vi "SetMotorType.vi"(0 "CmdLib In":refnum<k24>, 5 "DeviceKey In":string, 7 "Motor":i32, 9 "Motor Type":i32(ring) items=["NoMotor", "Undefined", "Tiny", "Standard"], 11 "error in (no error)":errorcluster) -> (4 "CmdLib Out":refnum<k24>, 8 "DeviceKey Out":string, 15 "error out":errorcluster)   [LabVIEW 2013]
uses:
  C:/Users/Saffmanlab/Documents/git/CsPyController/labview/cesium_controller/PicoMotor/NewFocus8742/CmdLib.dll
  CmdLib.dll
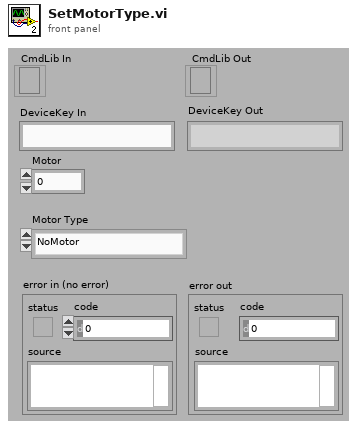
[diagram p1: front panel]
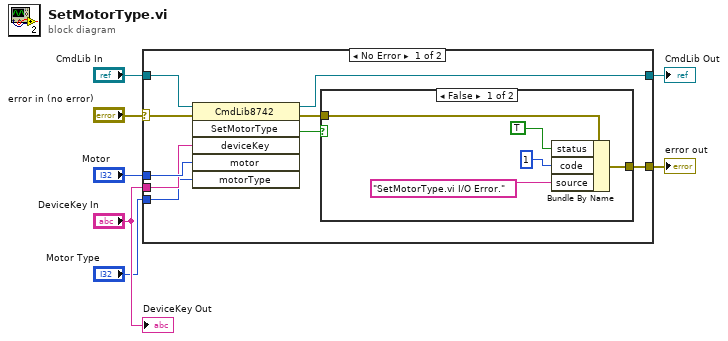
[diagram p0: block diagram]
diagram:
  n1 = case shown="No Error" "error in (no error)" {
    selector: "error in (no error)" -> [w12 w23]
    tunnel: "CmdLib In" -> [w16 w24]
    tunnel: [w15 w24] -> w6
    tunnel: "Motor" -> [w14 _]
    tunnel: "DeviceKey In" -> [w13 _]
    tunnel: [w9 w23] -> w3
    tunnel: "Motor Type" -> [w8 _]
    frame No Error {
      n2 = invoke class="CmdLib8742" method="SetMotorType"(reference=w16, error in=w12, "deviceKey"=w13, "motor"=w14, "motorType"=w8) -> (reference out=w15:refnum<k24>, error out=w10:errorcluster, "SetMotorType"=w11:bool)  [unwired: 1 in, 3 out]
      n3 = case shown="False" w11 {
        tunnel: w10 -> [w21 w22]
        tunnel: [w20 w22] -> w9
        frame False {
          n4 = Bundle By Name(cluster=w21, "status"=TRUE, "code"=1, "source"="SetMotorType.vi I/O Error.") -> (w20:errorcluster)
        }
        frame True {
        }
      }
    }
    frame Error {
    }
  }
  "error out" <- w3
  "CmdLib Out" <- w6
  "DeviceKey Out" <- "DeviceKey In"
